vi "Compute Roughness Params No Peak Density.vi"(0 "lower limit (0)":dbl, 1 "upper limit (5)":dbl=5.0, 2 "Video Frame":refnum<class "Video Frame.lvclass">, 3 "SubSampling Interval (10)":i32=10, 4 "Full? (T)":bool=TRUE) -> (5 "Roughness Parameters":T1)   [LabVIEW 2018]
uses:
  Classes/Video Frame/Video Frame.lvclass
  Roughness Parameters STYP.ctl
  1dfc503e-7255-4174-9bd2-c67dc4c7d3dc.vi
  aa907405-fc74-4412-a48d-6d9d57e3d258.vi
  04dbe17e-d004-441d-8831-1885748c1c99.vi
  aa907405-fc74-4412-a48d-6d9d57e3d258.vi/6f7a91ff-c696-4129-ae22-11c79f61275e.vi
  Classes/Roughness Averager/Roughness Averager.lvclass
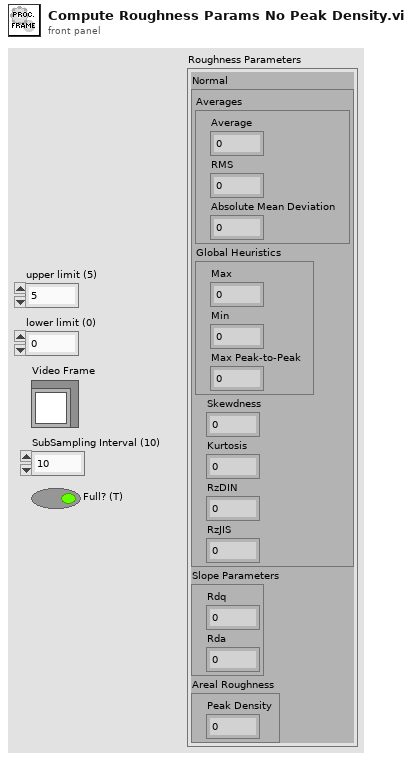
[diagram p1: front panel]
types:
  T1 = typedef "Roughness Parameters STYP.ctl" = cluster{"Normal":cluster{"Averages":cluster{"Average":dbl, "RMS":dbl, "Absolute Mean Deviation":dbl}, "Global Heuristics":cluster{"Max":dbl, "Min":dbl, "Max Peak-to-Peak":dbl}, "Skewdness":dbl, "Kurtosis":dbl, "RzDIN":dbl, "RzJIS":dbl}, "Slope Parameters":cluster{"Rdq":dbl, "Rda":dbl}, "Areal Roughness":cluster{"Peak Density":dbl}}
  T2 = typedef "IMAQ Image.ctl" = refnum<image>
  T3 = cluster{"Normal":cluster{"Averages":cluster{"Average":dbl, "RMS":dbl, "Absolute Mean Deviation":dbl}, "Global Heuristics":cluster{"Max":dbl, "Min":dbl, "Max Peak-to-Peak":dbl}, "Skewdness":dbl, "Kurtosis":dbl, "RzDIN":dbl, "RzJIS":dbl}, "Slope Parameters":cluster{"Rdq":dbl, "Rda":dbl}, "Areal Roughness":cluster{"Peak Density":dbl}}
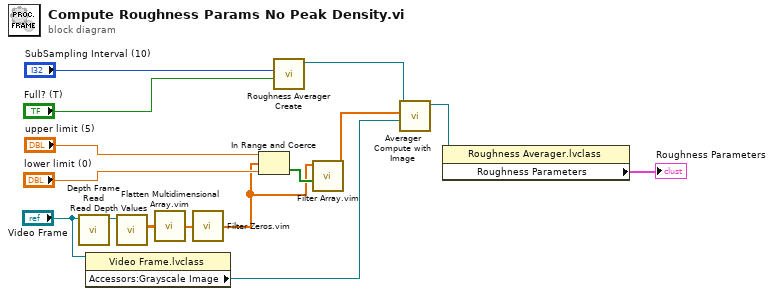
[diagram p0: block diagram]
diagram:
  n1 = call-dynamic "Depth Frame Read.vi"("Video Frame in"="Video Frame") -> ("Video Frame out"=w4:refnum<class "Video Frame.lvclass">)  [unwired: 6 in, 4 out]
  n2 = property class="Video Frame.lvclass"(reference="Video Frame") -> ("Accessors:Grayscale Image"=w11:T2)  [unwired: 1 in, 2 out]
  n3 = call-dynamic "Read Depth Values.vi"("Video Frame in"=w4) -> ("Depth Values"=w2:dbl[][])  [unwired: 8 in, 2 out]
  n4 = call "Flatten Multidimensional Array.vim"("Array"=w2) -> ("output array"=w3:dbl[])  [unwired: 14 in]
  n5 = call "Filter Zeros.vim"("Array"=w3) -> ("Array Out"=w1:dbl[])  [unwired: 14 in]
  n6 = In Range and Coerce(upper limit="upper limit (5)", x=w1, lower limit="lower limit (0)") -> (In Range?=w6:bool[])  [unwired: 1 out]
  n7 = call "Roughness Averager Create.vi"("Full? (T)"="Full? (T)", "SubSampling Interval (10)"="SubSampling Interval (10)") -> ("Roughness Averager out"=w13:refnum<class "Roughness Averager.lvclass">)  [unwired: 8 in, 1 out]
  n8 = call "Filter Array.vim"("Boolean Filter"=w6, "Array"=w1) -> ("Array Out"=w5:dbl[])  [unwired: 9 in]
  n9 = call-dynamic "Averager Compute with Image.vi"("Grayscale Image"=w11, "Data"=w5, "Roughness Averager in"=w13) -> ("Roughness Averager out"=w10:refnum<class "Roughness Averager.lvclass">)  [unwired: 7 in, 1 out]
  n10 = property class="Roughness Averager.lvclass"(reference=w10) -> ("Roughness Parameters"=→"Roughness Parameters":T3)  [unwired: 1 in, 2 out]
